vi "DANTE init & config.vi"(8 "Boards to configure":u8(slide) scale=0.0..8.0, 9 "DPP Configuration":T1={"reset_recovery_time"=300, "edge_peaking_time"=4, "flat_top"=7, "peaking_time"=32, "gain"=1.0, "max_risetime"=0.0, "fast_filter_thr"=45, "zero_peak_freq"=1.0, "inverted_input"=0, "base_offset"=0, "reset_threshold"=1000, "overflow_recovery"=30, "tail_coefficient"=0.0, "energy_filter_thr"=23, "energy_baseline_thr"=23, "max_peaking_time"=35, "edge_flat_top"=7, "time_constant"=0.0, "baseline_samples"=64, "other_param"=0}, 10 "Number of boards in chain":u8(slide)=1 scale=1.0..8.0, 11 "IP Address":string="10.96.0.110") -> (0 "DANTE configured":bool, 1 "DANTE loaded":bool, 2 "IP added":bool, 3 "Library Initialized":bool, 5 "identifier out":string)   [LabVIEW 2015]
uses:
  libs/XGL_DPP.lvlib
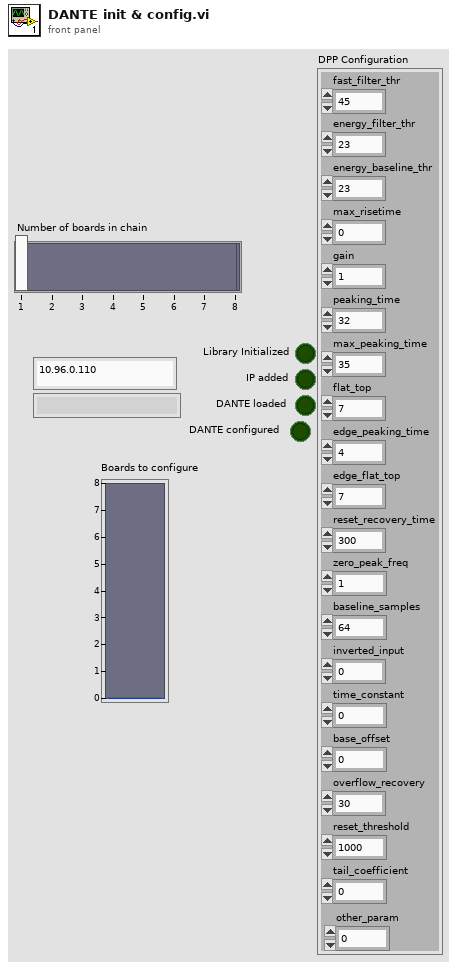
[diagram p1: front panel]
types:
  T1 = cluster{"reset_recovery_time":u32, "edge_peaking_time":u32, "flat_top":u32, "peaking_time":u32, "gain":dbl, "max_risetime":dbl, "fast_filter_thr":u32, "zero_peak_freq":dbl, "inverted_input":u8, "base_offset":u32, "reset_threshold":u32, "overflow_recovery":u32, "tail_coefficient":dbl, "energy_filter_thr":u32, "energy_baseline_thr":u32, "max_peaking_time":u32, "edge_flat_top":u32, "time_constant":dbl, "baseline_samples":u32, "other_param":u32}
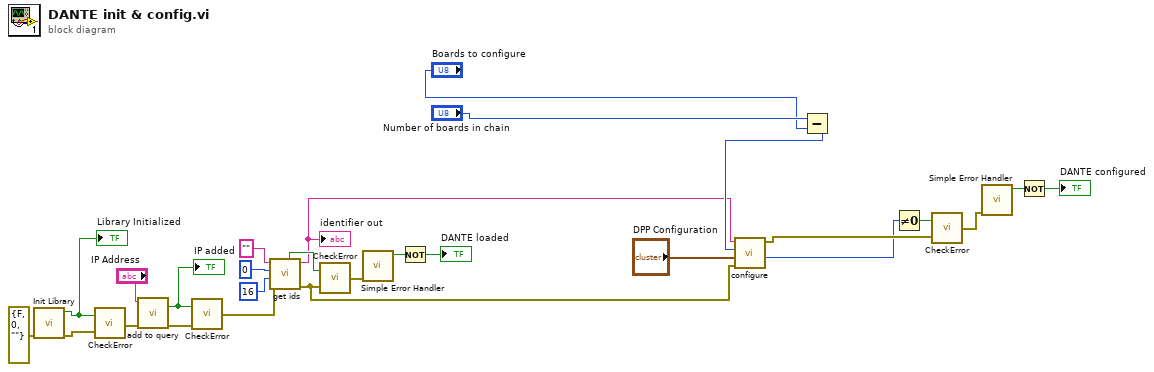
[diagram p0: block diagram]
diagram:
  n1 = call "Init Library.vi"("error in (no error)"=errorcluster {"status"=FALSE, "code"=0, "source"=""}) -> ("error out"=w14:errorcluster, "function return"=w15:bool)  [unwired: 9 in]
  "Library Initialized" <- w15
  n2 = call "CheckError.vi"("error in (no error)"=w14, "ret_val"=w15) -> ("error out"=w16:errorcluster)
  n3 = call "add to query.vi"("error in (no error)"=w16, "address"="IP Address") -> ("error out"=w18:errorcluster, "function return"=w19:bool)  [unwired: 7 in, 1 out]
  "IP added" <- w19
  n4 = call "CheckError.vi"("error in (no error)"=w18, "ret_val"=w19) -> ("error out"=w24:errorcluster)
  n5 = call "get ids.vi"("error in (no error)"=w24, "id_size"=u32 16 ("char_size"), "nb"=u32 0, "identifier"="") -> ("error out"=w5:errorcluster, "identifier out"=w6:string, "function return"=w21:bool)  [unwired: 3 in, 2 out]
  "identifier out" <- w6
  n6 = call "CheckError.vi"("error in (no error)"=w5, "ret_val"=w21) -> ("error out"=w25:errorcluster)
  n7 = call <vilib>:"Simple Error Handler.vi"("error in (no error)"=w25) -> ("error?"=w26:bool)  [unwired: 4 in, 4 out]
  n8 = Not(x=w26) -> (.not. x?=→"DANTE loaded":bool)
  n9 = Subtract(x="Number of boards in chain", y="Boards to configure") -> (x-y=w11:u8)
  n10 = call "configure.vi"("error in (no error)"=w5, "DPP Configuration"="DPP Configuration", "Board"=w11, "identifier"=w6) -> ("function return"=w9:u32, "error out"=w10:errorcluster)  [unwired: 2 in]
  n11 = Not Equal To 0?(x=w9) -> (x != 0?=w12:bool)
  n12 = call "CheckError.vi"("error in (no error)"=w10, "ret_val"=w12) -> ("error out"=w2:errorcluster)
  n13 = call <vilib>:"Simple Error Handler.vi"("error in (no error)"=w2) -> ("error?"=w3:bool)  [unwired: 4 in, 4 out]
  n14 = Not(x=w3) -> (.not. x?=→"DANTE configured":bool)
